vi "Tiles indicator.vi"(7 "Actions":T1=enum."Clear", 8 "Error In":errorcluster, 10 "# tiles":u32, 11 "# X tiles":u32) -> (0 "Error Out":errorcluster, 1 "# tiles":u32, 2 "# Y tiles":u32, 3 "# X tiles":u32)   [LabVIEW 2018]
uses:
  Controls/FGV Actions.ctl
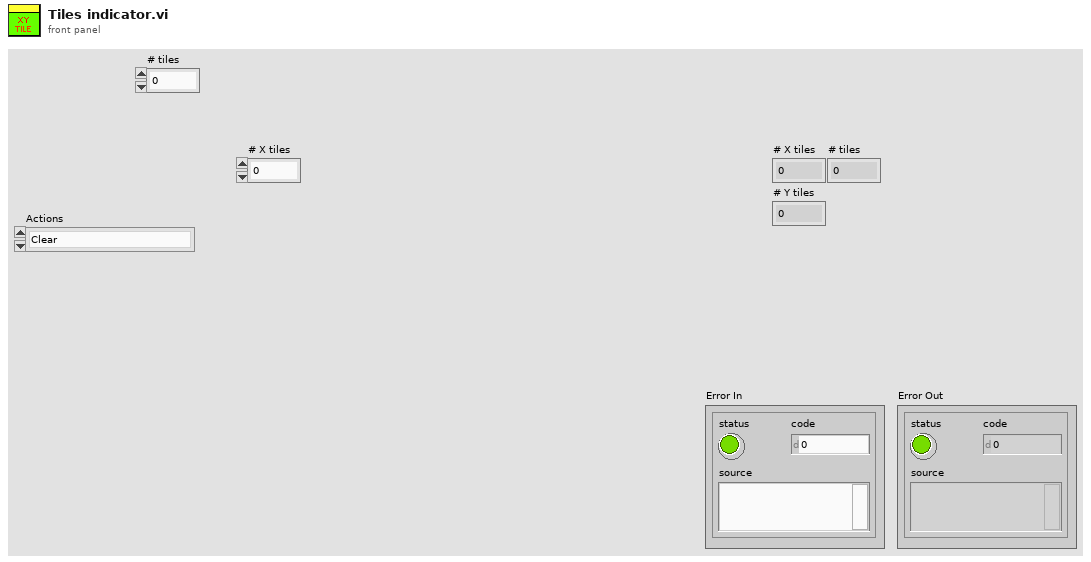
[diagram p1: front panel]
types:
  T1 = typedef "FGV Actions.ctl" = enum16{"Init", "Set", "Get", "Clear"}
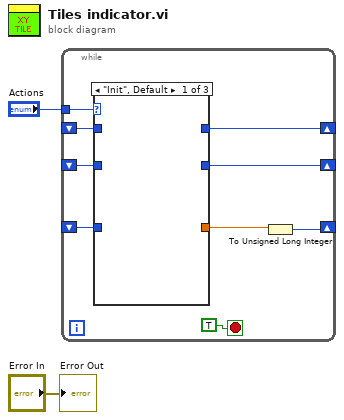
[diagram p0: block diagram]
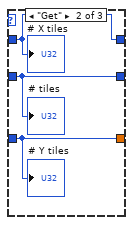
[diagram p2: hidden frame]
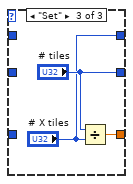
[diagram p3: hidden frame]
diagram:
  n1 = while {
    shift-right: [w11] -> _
    shift-left: _ -> [w9]
    tunnel: "Actions" -> [w10]
    shift-right: [w7] -> _
    shift-left: _ -> [w6]
    shift-right: [w3] -> _
    shift-left: _ -> [w5]
    stop <- TRUE stop-if-true
    n2 = case shown="\"Init\", Default" w10 {
      tunnel: [_ w14 "# X tiles"] -> w11
      tunnel: w9 -> [_ w14 _]
      tunnel: [_ w13 "# tiles"] -> w7
      tunnel: w6 -> [_ w13 _]
      tunnel: [_ w12 w15] -> w4
      tunnel: w5 -> [_ w12 _]
      frame "Init", Default {
      }
      frame "Get" {
        "# X tiles" <- w14
        "# tiles" <- w13
        "# Y tiles" <- w12
      }
      frame "Set" {
        n3 = Divide(x="# tiles", y="# X tiles") -> (x/y=w15:dbl)
      }
    }
    n4 = To Unsigned Long Integer(number=w4) -> (unsigned 32bit integer=w3:u32)
  }
  "Error Out" <- "Error In"
